vi "ElapsedTimeFGV.vi"(7 "Timer  Mode":enum16{"Reset", "Read Status", "Set Auto Reset"}(ring), 8 "Error In":errorcluster, 9 "Auto Reset (F)":bool, 11 "Time Limit (s)":dbl) -> (0 "Error Out":errorcluster, 1 "Time left(s)":string, 2 "Time left (s)":dbl, 3 "Time Has Elapsed":bool)   [LabVIEW 2020]
doc: "This SubVI is an FGV that wraps the express VI. By default the FGV reset puts False in the auto reset input (and shift register). This occurs only when the \"Set Auto Reset\" case is used. The auto reset must be set as a separate call to the FGV."
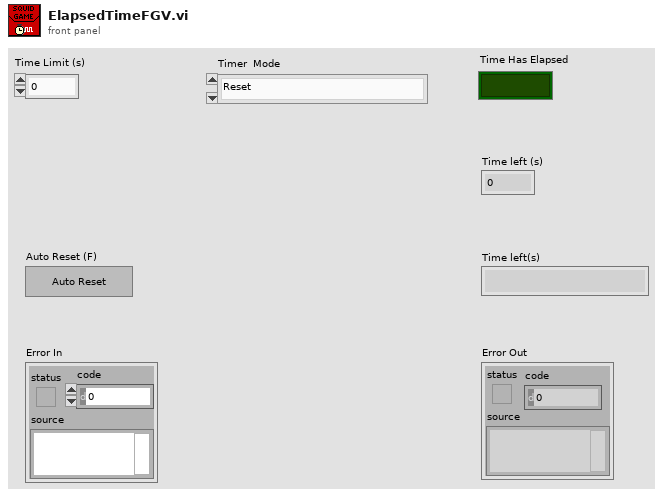
[diagram p1: front panel]
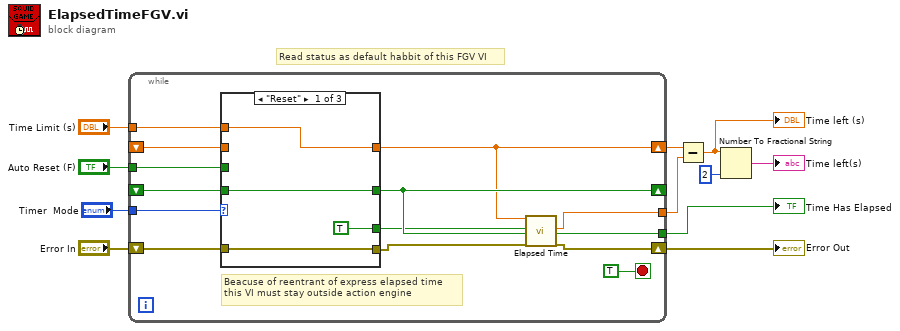
[diagram p0: block diagram]
diagram:
  # "Read status as default habbit of this FGV VI"
  n1 = while {
    tunnel: "Timer  Mode" -> [w24]
    shift-right: [w16] -> w7
    shift-left: "Error In" -> [w23]
    shift-right: [w20] -> _
    shift-left: _ -> [w21]
    tunnel: "Auto Reset (F)" -> [w22]
    tunnel: "Time Limit (s)" -> [w19]
    shift-right: [w18] -> w2
    shift-left: _ -> [w14]
    tunnel: [w13] -> w6
    tunnel: [w12] -> w1
    stop <- TRUE stop-if-true
    # "Beacuse of reentrant of express elapsed time \nthis VI must stay outside action engine"
    n2 = case shown="\"Reset\"" w24 {
      tunnel: w23 -> [w28 w30 w33]
      tunnel: [w26 w32 w35] -> w20
      tunnel: w22 -> [_ _ w35]
      tunnel: w21 -> [w26 w32 _]
      tunnel: w19 -> [w29 _ _]
      tunnel: [w29 w31 w34] -> w18
      tunnel: [w28 w30 w33] -> w17
      tunnel: [TRUE _ _] -> w15
      tunnel: w14 -> [_ w31 w34]
      frame "Reset" {
      }
      frame "Read Status", Default {
        # "No reset"
      }
      frame "Set Auto Reset" {
        # "No reset"
      }
    }
    n3 = call "Elapsed Time"("Time Target (s)"=w18, "Reset"=w15, "Auto Reset"=w20, "error in (no error)"=w17) -> ("Elapsed Time (s)"=w12:dbl, "Time has Elapsed"=w13:bool, "error out"=w16:errorcluster)  [unwired: 8 in, 5 out]
  }
  "Error Out" <- w7
  "Time Has Elapsed" <- w6
  n4 = Subtract(x=w2, y=w1) -> (x-y=w3:dbl)
  "Time left (s)" <- w3
  n5 = Number To Fractional String(number=w3, precision (6)=i16 2) -> (F-format string=→"Time left(s)":string)  [unwired: 2 in]
